vi "Get Scanner.vi"(8 "error in (no error)":errorcluster, 11 "Magnet in":refnum<class "Magnet.lvclass">) -> (0 "error out":errorcluster, 2 "Default Scanner out":refnum<class "Scanner.lvclass">)   [LabVIEW 2009, in "Magnet.lvclass"]
doc: "(Dynamic) Returns the default Scanner object that scans over this Scannable. (Note that a Scannable may have multiple Scanners associated with it.) A Scanner is an analogue to an Iterator class in other languages."
uses:
  Magnet.lvclass
  Scanners/Scanner/Scanner.lvclass
  Scans/Magnetic Field/Magnetic Field.lvclass
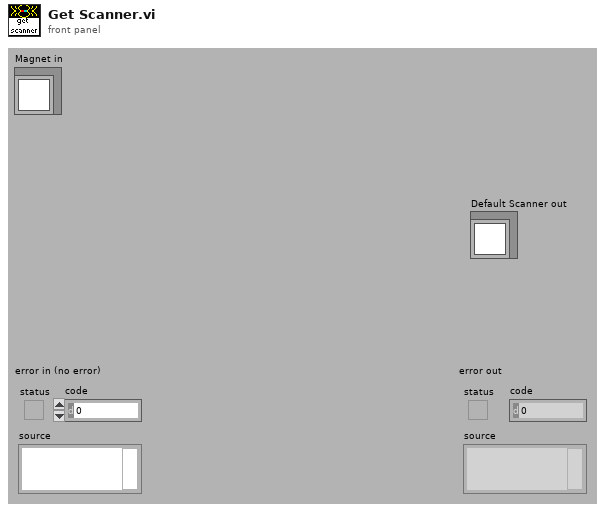
[diagram p1: front panel]
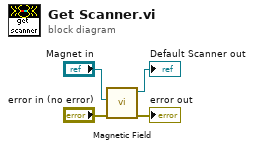
[diagram p0: block diagram]
diagram:
  n1 = call "Magnetic Field.vi"("error in (no error)"="error in (no error)", "Magnet in"="Magnet in") -> ("error out"=→"error out":errorcluster, "Magnetic Field.lvclass out"=→"Default Scanner out":refnum<class "Magnetic Field.lvclass">)  [unwired: 8 out]
